vi "Device Initialization.vi"(8 "에러 입력(에러 없음)":errorcluster, 9 "VISA Resource Name":string, 11 "Channel Ref":T1 format="%.0x") -> (0 "에러 출력":errorcluster)   [LabVIEW 2017, in "Serial Communcation Devices Custom Device.lvlib"]
uses:
  Serial Communcation Devices Custom Device.lvlib
  <vilib>/NI Veristand/Custom Device API/Custom Device Item Ref.ctl
  <vilib>/NI Veristand/Custom Device API/Set Item Property (Boolean).vi
  <vilib>/NI Veristand/Custom Device API/Set Item Property (U16).vi
  <vilib>/NI Veristand/Custom Device API/Set Item Property (String).vi
  <vilib>/NI Veristand/Custom Device API/Custom Device API.lvlib
panel:
  out "Channel Ref Out":T1 format="%.0x"
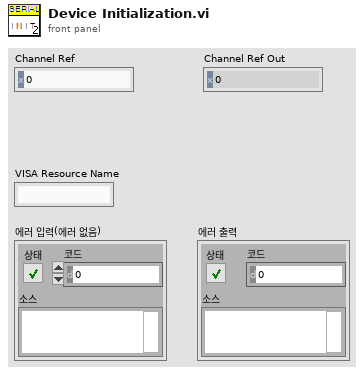
[diagram p1: front panel]
types:
  T1 = typedef "Custom Device API.lvlib/Custom Device Item Ref.ctl" = u64
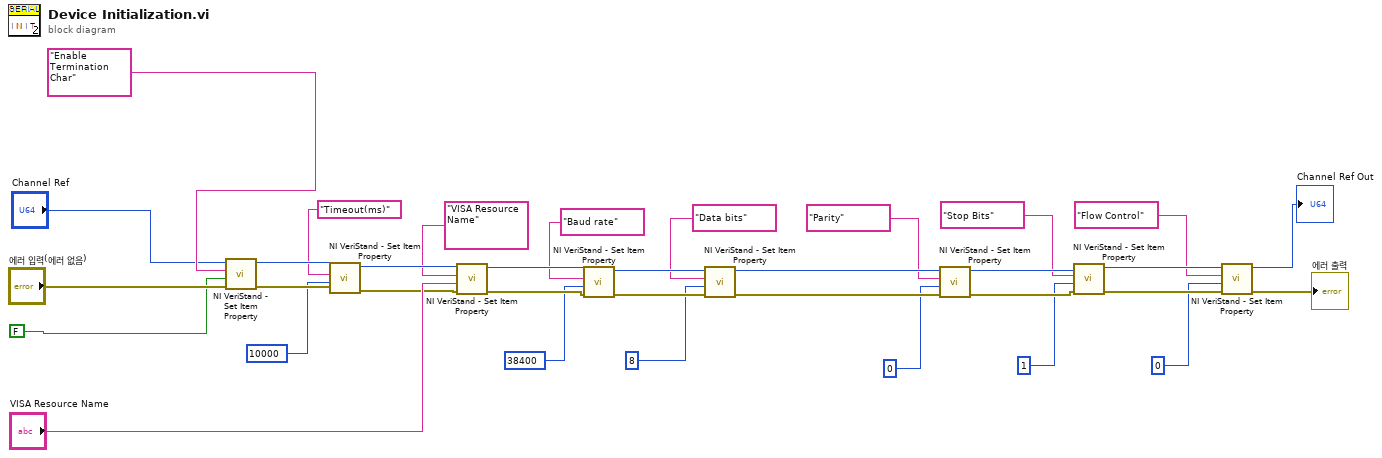
[diagram p0: block diagram]
diagram:
  n1 = call-poly <vilib>:"NI VeriStand - Set Item Property.vi"("error in (no error)"="에러 입력(에러 없음)", "Value"=FALSE, "Property Name"="Enable Termination Char", "Item Ref in"="Channel Ref") -> ("error out"=w20:errorcluster, "Item Ref out"=w27:T1)  [unwired: 5 in, 1 out]
  n2 = call-poly <vilib>:"NI VeriStand - Set Item Property.vi"("error in (no error)"=w20, "Value"=10000, "Property Name"="Timeout(ms)", "Item Ref in"=w27) -> ("error out"=w21:errorcluster, "Item Ref out"=w28:T1)  [unwired: 5 in, 1 out]
  n3 = call-poly <vilib>:"NI VeriStand - Set Item Property.vi"("error in (no error)"=w21, "Value"="VISA Resource Name", "Property Name"="VISA Resource Name", "Item Ref in"=w28) -> ("error out"=w22:errorcluster, "Item Ref out"=w29:T1)  [unwired: 5 in, 1 out]
  n4 = call-poly <vilib>:"NI VeriStand - Set Item Property.vi"("error in (no error)"=w22, "Value"=38400, "Property Name"="Baud rate", "Item Ref in"=w29) -> ("error out"=w23:errorcluster, "Item Ref out"=w30:T1)  [unwired: 5 in, 1 out]
  n5 = call-poly <vilib>:"NI VeriStand - Set Item Property.vi"("error in (no error)"=w23, "Value"=8, "Property Name"="Data bits", "Item Ref in"=w30) -> ("error out"=w24:errorcluster, "Item Ref out"=w16:T1)  [unwired: 5 in, 1 out]
  n6 = call-poly <vilib>:"NI VeriStand - Set Item Property.vi"("error in (no error)"=w24, "Value"=0, "Property Name"="Parity", "Item Ref in"=w16) -> ("error out"=w25:errorcluster, "Item Ref out"=w17:T1)  [unwired: 5 in, 1 out]
  n7 = call-poly <vilib>:"NI VeriStand - Set Item Property.vi"("error in (no error)"=w25, "Value"=1, "Property Name"="Stop Bits", "Item Ref in"=w17) -> ("error out"=w26:errorcluster, "Item Ref out"=w18:T1)  [unwired: 5 in, 1 out]
  n8 = call-poly <vilib>:"NI VeriStand - Set Item Property.vi"("error in (no error)"=w26, "Value"=0, "Property Name"="Flow Control", "Item Ref in"=w18) -> ("error out"=→"에러 출력":errorcluster, "Item Ref out"=→"Channel Ref Out":T1)  [unwired: 5 in, 1 out]
